vi "Waveform - Align Timestamps.vi"() -> ()   [LabVIEW 2020]
doc: "Shows how to replace all the timestamp values with the value of the index element in the array."
uses:
  <vilib>/Waveform/WDTOps.llb/WDT Align Waveform Timestamps DBL.vi
panel:
  out "After Timestamps Aligned":waveform(dbl)[](graph)
  in  "Index":i32 min=0 max=2 step=1
  out "Before Timestamps Aligned":waveform(dbl)[](graph)
  # "Overview: Demonstrates how to align the timestamps of different waveforms with the Align Waveform Timestamps VI.\nInstructions:\n1. Select an Index value to specify which waveform's initial timestamp to use. \n2. Run the VI. The timestamp of the waveform at the specified Index will be used as the new timestamp for all the waveforms."
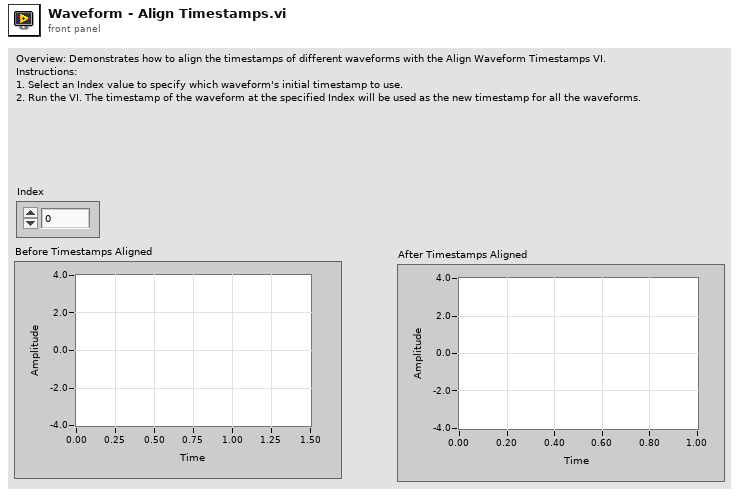
[diagram p1: front panel]
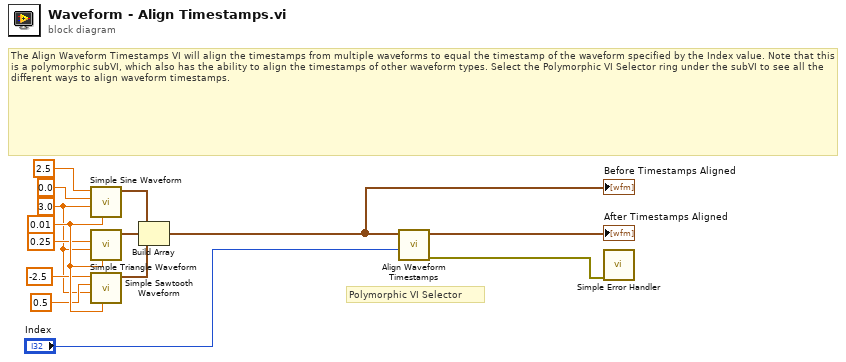
[diagram p0: block diagram]
diagram:
  w12 = 0.01
  w8 = 3.0
  # "The Align Waveform Timestamps VI will align the timestamps from multiple waveforms to equal the timestamp of the waveform specified by the Index value. Note that this is a polymorphic subVI, which also has the ability to align the timestamps of other waveform types. Select the Polymorphic VI Selector ring under the subVI to see all the different ways to align waveform timestamps."
  # "Polymorphic VI Selector"
  n1 = call "Simple Sine Waveform.vi"("delta t"=w12, "n cycles"=w8, "t0"=0.0, "offset"=2.5) -> ("sine waveform"=w4:waveform(dbl))  [unwired: 7 in]
  n2 = call "Simple Triangle Waveform.vi"("delta t"=w12, "n cycles"=w8, "t0"=0.25) -> ("triangle waveform"=w5:waveform(dbl))  [unwired: 8 in]
  n3 = call "Simple Sawtooth Waveform.vi"("delta t"=w12, "n cycles"=w8, "t0"=0.5, "offset"=-2.5) -> ("sawtooth waveform"=w6:waveform(dbl))  [unwired: 7 in]
  n4 = Build Array(w4, w5, w6) -> (w2:waveform(dbl)[])
  "Before Timestamps Aligned" <- w2
  n5 = call-poly <vilib>:"Align Waveform Timestamps.vi"("index"="Index", "waveforms in"=w2) -> ("error out"=w13:errorcluster, "waveforms out"=→"After Timestamps Aligned":waveform(dbl)[])  [unwired: 8 in]
  n6 = call <vilib>:"Simple Error Handler.vi"("error in (no error)"=w13) -> ()  [unwired: 4 in, 5 out]
